vi "test_findAllPollers.vi"() -> ()   [LabVIEW 2011, in "ttmServer.lvclass"]
uses:
  ttmServer.lvclass
panel:
  out "pollerFileNames":string[](array[string])
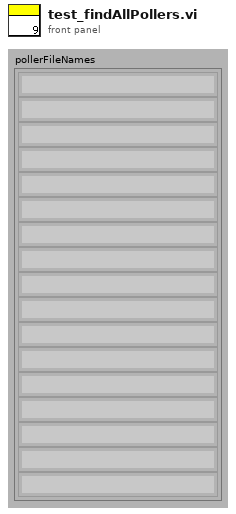
[diagram p1: front panel]
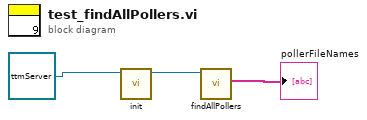
[diagram p0: block diagram]
diagram:
  n1 = call "init.vi"("ttm_poller_panel.vi.lvclass"=refnum<class "ttmServer.lvclass"> refnum) -> ("output cluster"=w1:refnum<class "ttmServer.lvclass">)  [unwired: 10 in]
  n2 = call "findAllPollers.vi"("ttm_poller_panel_in"=w1) -> ("pollerFileNames"=→"pollerFileNames":string[])  [unwired: 9 in, 1 out]
